vi "IB_RW_Project_RegData.vi"(7 "action":T3, 8 "error in (no error)":errorcluster, 9 "index in":string, 10 "RegData":T2, 11 "buildObject":T1) -> (0 "error out":errorcluster, 1 "index out":string, 2 "RegData":T2, 3 "buildObject out":T1)   [LabVIEW 2020]
doc: "Reads and writes the data to the object property bag."
uses:
  <resource>/Framework/Providers/API/ItemRef.ctl
  <vilib>/AppBuilder/IB_RW_Project/IB_RW_Project_RegData_Data.ctl
  <vilib>/AppBuilder/IB_RW_Project/IB_RW_Project_PropBag_Action.ctl
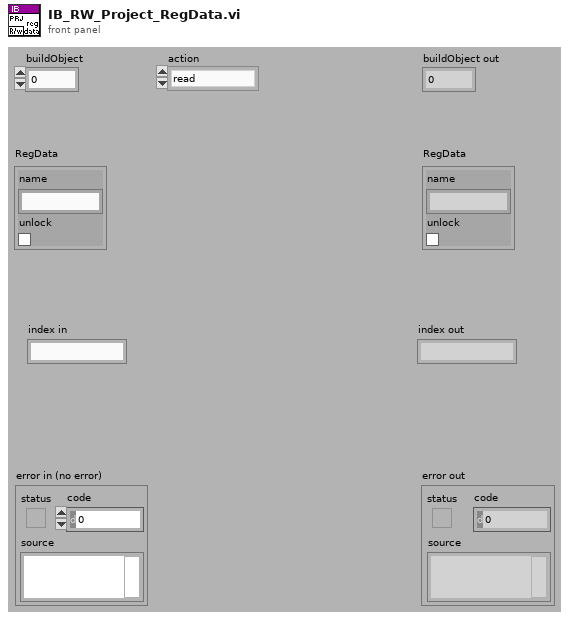
[diagram p1: front panel]
types:
  T1 = typedef "ItemRef.ctl" = u64
  T2 = typedef "IB_RW_Project_RegData_Data.ctl" = cluster{"name":string, "unlock":bool}
  T3 = typedef "IB_RW_Project_PropBag_Action.ctl" = enum16{"read", "write", "clear", "readPrevious", "writePrevious", "clearPrevious"}
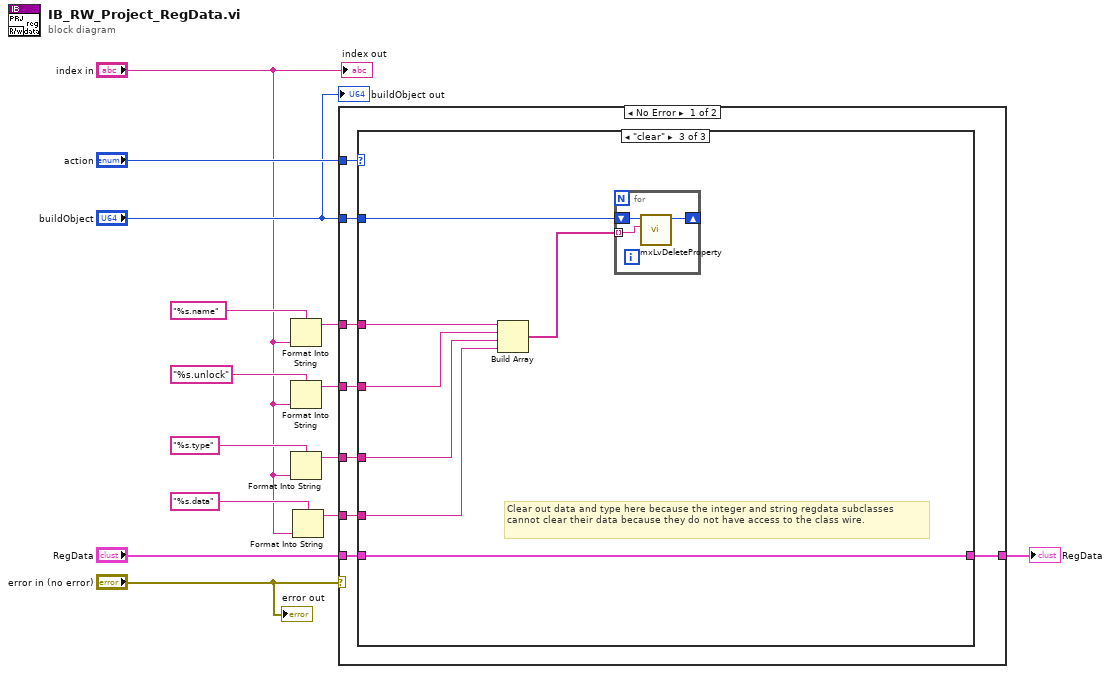
[diagram p0: block diagram]
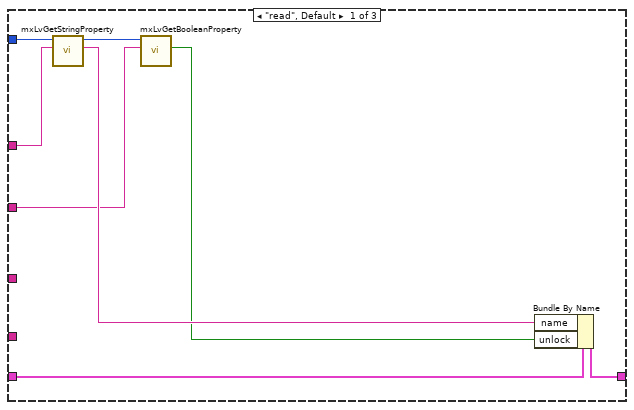
[diagram p2: hidden frame]
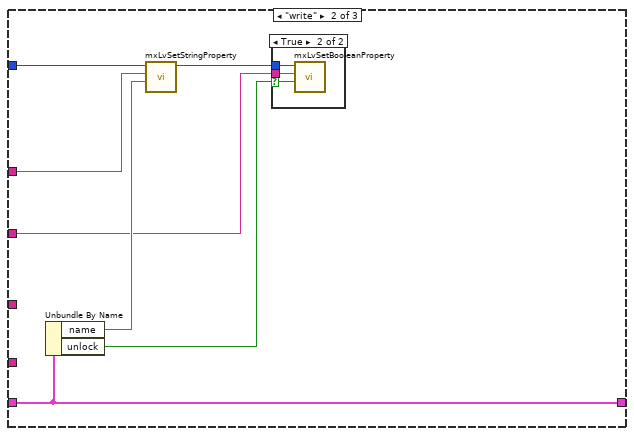
[diagram p3: hidden frame]
diagram:
  n1 = Format Into String(format string="%s.name", "index in") -> (resulting string=w11:string)  [unwired: 2 in, 1 out]
  n2 = Format Into String(format string="%s.unlock", "index in") -> (resulting string=w6:string)  [unwired: 2 in, 1 out]
  n3 = Format Into String(format string="%s.type", "index in") -> (resulting string=w4:string)  [unwired: 2 in, 1 out]
  n4 = Format Into String(format string="%s.data", "index in") -> (resulting string=w1:string)  [unwired: 2 in, 1 out]
  n5 = case shown="No Error" "error in (no error)" {
    tunnel: "action" -> [w22 _]
    tunnel: "RegData" -> [w21 w51]
    tunnel: w11 -> [w20 _]
    tunnel: w6 -> [w19 _]
    tunnel: [w18 w51] -> w10
    tunnel: "buildObject" -> [w17 _]
    tunnel: w4 -> [w16 _]
    tunnel: w1 -> [w15 _]
    frame No Error {
      n6 = case shown="\"clear\"" w22 {
        tunnel: w17 -> [w28 w36 w45]
        tunnel: w21 -> [w30 w37 w47]
        tunnel: w20 -> [w27 w35 w46]
        tunnel: w19 -> [w25 w33 w43]
        tunnel: [w29 w37 w47] -> w18
        tunnel: w16 -> [_ _ w42]
        tunnel: w15 -> [_ _ w41]
        frame "read", Default {
          n7 = call <resource>:"mxLvGetStringProperty.vi"("Tag"=w27, "Item"=w28) -> ("Value"=w26:string, "Item"=w24:T1)  [unwired: 1 in, 7 out]
          n8 = call <resource>:"mxLvGetBooleanProperty.vi"("Tag"=w25, "Item"=w24) -> ("Value"=w23:bool)  [unwired: 1 in, 8 out]
          n9 = Bundle By Name(cluster=w30, "name"=w26, "unlock"=w23) -> (w29:T2)
        }
        frame "write" {
          n10 = Unbundle By Name(w37) -> ("name"=w34:string, "unlock"=w32:bool)
          n11 = call <resource>:"mxLvSetStringProperty.vi"("Value (\"\")"=w34, "Tag"=w35, "Item"=w36) -> ("Item"=w31:T1)  [unwired: 2 in, 6 out]
          n12 = case shown="True" w32 {
            selector: w32 -> [_ w38]
            tunnel: w31 -> [_ w40]
            tunnel: w33 -> [_ w39]
            frame False {
            }
            frame True {
              n13 = call <resource>:"mxLvSetBooleanProperty.vi"("Value (F)"=w38, "Tag"=w39, "Item"=w40) -> ()  [unwired: 2 in, 7 out]
            }
          }
        }
        frame "clear" {
          # "Clear out data and type here because the integer and string regdata subclasses cannot clear their data because they do not have access to the class wire."
          n14 = Build Array(w46, w43, w42, w41) -> (w44:string[])
          n15 = for {
            shift-right: [w50] -> _
            shift-left: w45 -> [w49]
            tunnel: w44 -> [w48] mode=indexing
            n16 = call <resource>:"mxLvDeleteProperty.vi"("Tag"=w48, "Item"=w49) -> ("Item"=w50:T1)  [unwired: 1 in, 8 out]
          }
        }
      }
    }
    frame Error {
    }
  }
  "RegData" <- w10
  "error out" <- "error in (no error)"
  "buildObject out" <- "buildObject"
  "index out" <- "index in"
